vi "Кнопка Следует за мышью.vi"() -> ()   [LabVIEW 2021]
panel:
  in  "stop":bool
  in  "Вкл":bool
  out "Ldb":bool
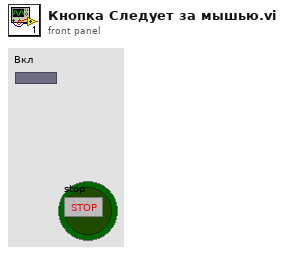
[diagram p1: front panel]
types:
  T1 = typedef "LVPoint32TypeDef.ctl" = cluster{"Horizontal":i32, "Vertical":i32}
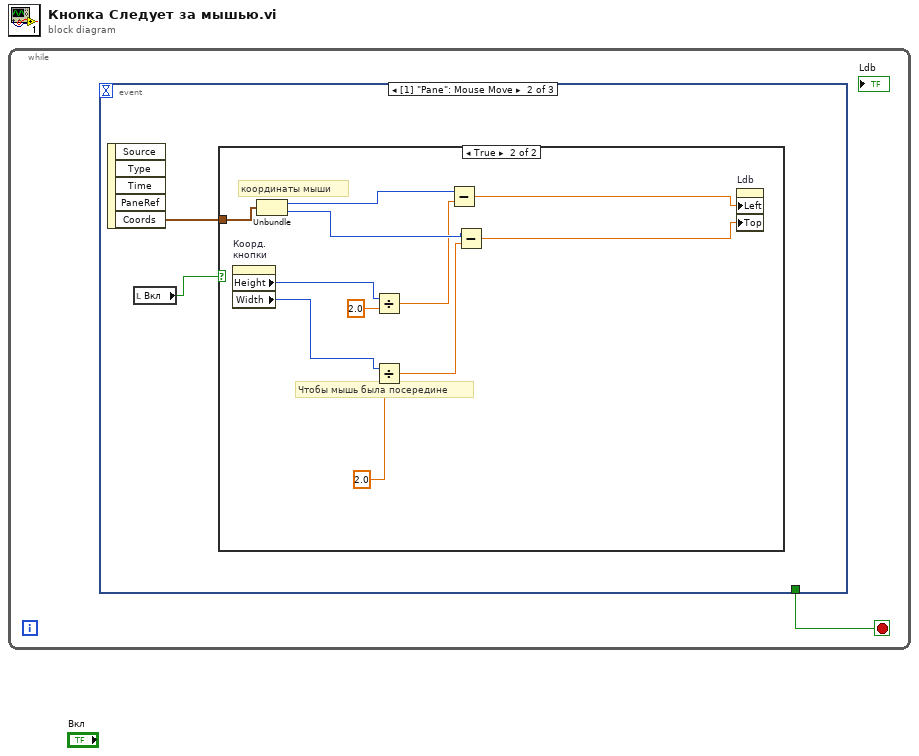
[diagram p0: block diagram]
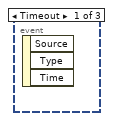
[diagram p2: hidden frame]
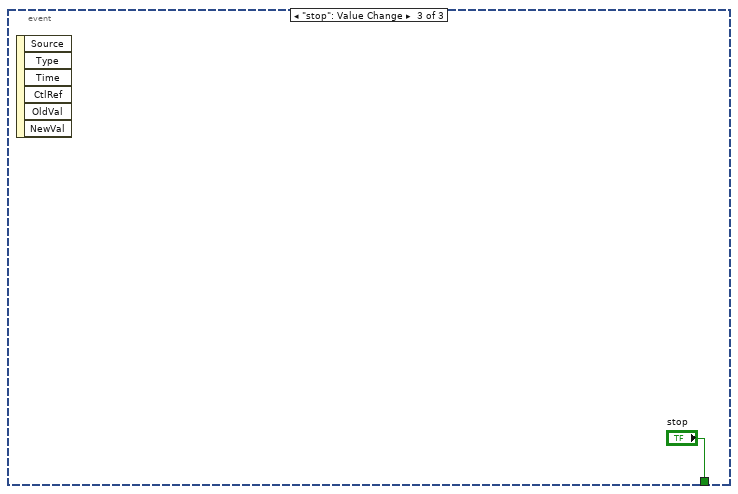
[diagram p4: hidden frame]
diagram:
  n1 = while {
    stop <- w1 stop-if-true
    n2 = event shown="[1] \"Pane\": Mouse Move" {
      selector: _ -> [_ _ _]
      dyn-events: _ -> [_ _ _]
      timeout: _ -> [_ _ _]
      tunnel: [_ _ "stop"] -> w1
      event Timeout {
        n3 = event-data() -> ()  [unwired: 1 in, 3 out]
      }
      event Mouse Move {
        n4 = event-data() -> ("Coords"=w3:T1)  [unwired: 1 in, 4 out]
        n5 = local read "Вкл"() -> (w2:bool)
        n6 = case shown="True" w2 {
          tunnel: w3 -> [_ w14]
          frame False {
          }
          frame True {
            # "Чтобы мышь была посередине"
            # "координаты мыши"
            n7 = property on="Коорд. \nкнопки" class="Bool (strict)"() -> ("Height"=w10:u32, "Width"=w11:u32)  [unwired: 2 in, 2 out]
            n8 = Unbundle(w14) -> ("Horizontal"=w9:i32, "Vertical"=w8:i32)
            n9 = Divide(x=w10, y=2.0) -> (x/y=w6:dbl)
            n10 = Divide(x=w11, y=2.0) -> (x/y=w7:dbl)
            n11 = Subtract(x=w9, y=w6) -> (x-y=w5:dbl)
            n12 = Subtract(x=w8, y=w7) -> (x-y=w4:dbl)
            n13 = property on="Ldb" class="Bool (strict)"("Left"=w5, "Top"=w4) -> ()  [unwired: 2 in, 2 out]
          }
        }
      }
      event "stop": Value Change {
        n14 = event-data() -> ()  [unwired: 1 in, 6 out]
      }
    }
  }
